vi "1553B-PACKET-1.vi"(8 "数组":u8[](array[numeric])) -> (5 "北向速度":i32, 6 "高度":i32, 7 "纬度":i32, 9 "经度":i32, 10 "系统状态":cluster{"工作状态":string, "工作模式":string}, 11 "真航向":i16, 12 "对准数据来源字":cluster{"位置数据":string, "姿态数据":string}, 13 "横滚角":i16, 14 "组合模式受控状态":cluster{"自动":bool, " 强选":bool}, 15 "俯仰角":i16, 16 "组合数据来源":T7, 17 "地向速度":i32, 18 "组合状态字":T6, 19 "东向速度":i32, 20 "组合导航数据有效字":T1, 21 "GPSBD辅助数据有效字":T5, 22 "系统故障字1":T2, 23 "GLOADSST辅助数据有效字":T4, 24 "北京时间":timestamp, 25 "惯组数据有效字":T3, 26 "单次上电工作时间":i32)   [LabVIEW 2012]
uses:
  index-i32.vi
  index-dbl.vi
  XX-I32.vi
  index-i16.vi
  XX-I16.vi
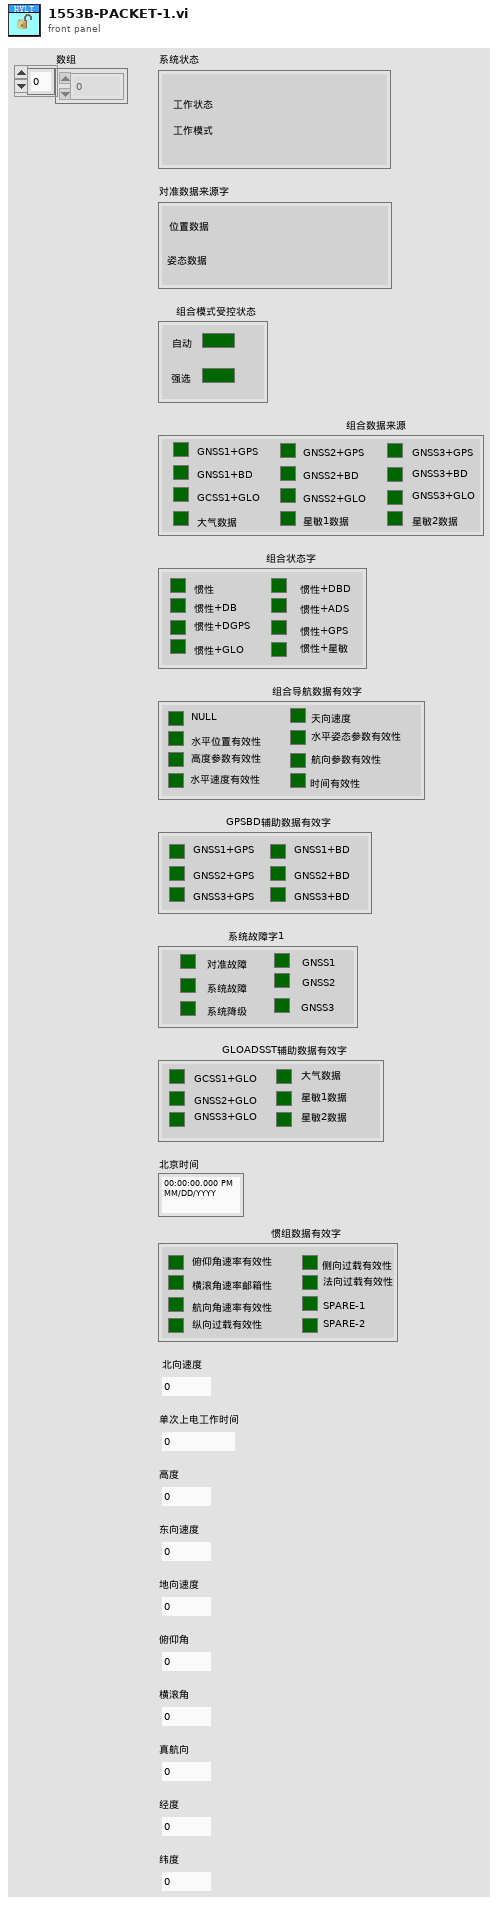
[diagram p1: front panel]
types:
  T1 = cluster{"水平姿态参数有效性":bool, "天向速度":bool, "水平速度有效性":bool, "高度参数有效性":bool, "水平位置有效性":bool, "NULL":bool, " 时间有效性":bool, "航向参数有效性":bool}
  T2 = cluster{"对准故障":bool, "系统故障":bool, "系统降级":bool, "GNSS1":bool, "GNSS2":bool, "GNSS3":bool}
  T3 = cluster{"法向过载有效性":bool, "侧向过载有效性":bool, "纵向过载有效性":bool, "航向角速率有效性":bool, "横滚角速率邮箱性":bool, "俯仰角速率有效性":bool, "SPARE-2":bool, "SPARE-1":bool}
  T4 = cluster{"GCSS1+GLO":bool, "GNSS2+GLO":bool, "GNSS3+GLO":bool, "大气数据":bool, "星敏1数据":bool, "星敏2数据":bool}
  T5 = cluster{"GNSS1+GPS":bool, "GNSS2+GPS":bool, "GNSS2+BD":bool, "GNSS3+BD":bool, "GNSS3+GPS":bool, "GNSS1+BD":bool}
  T6 = cluster{"惯性":bool, "惯性+DGPS":bool, "惯性+DBD":bool, "惯性+GPS":bool, "惯性+DB":bool, "惯性+GLO":bool, "惯性+ADS":bool, "惯性+星敏":bool}
  T7 = cluster{"GNSS1+GPS":bool, "GNSS1+BD":bool, "GCSS1+GLO":bool, "GNSS3+GPS":bool, "GNSS2+GPS":bool, "GNSS2+BD":bool, "GNSS2+GLO":bool, "GNSS3+BD":bool, "GNSS3+GLO":bool, "星敏1数据":bool, "星敏2数据":bool, "大气数据":bool}
  T8 = cluster{"NULL":bool, "水平位置有效性":bool, "高度参数有效性":bool, "水平速度有效性":bool, "天向速度":bool, "水平姿态参数有效性":bool, " 时间有效性":bool, "航向参数有效性":bool}
  T9 = cluster{"俯仰角速率有效性":bool, "横滚角速率邮箱性":bool, "航向角速率有效性":bool, "纵向过载有效性":bool, "侧向过载有效性":bool, "法向过载有效性":bool, "SPARE-2":bool, "SPARE-1":bool}
  T10 = cluster{"GNSS1+GPS":bool, "GNSS1BD":bool, "GNSS3+GPS":bool, "GNSS2+GPS":bool, "GNSS2BD":bool, "GNSS3BD":bool}
  T11 = cluster{"GNSS1+GPS":bool, "GNSS1BD":bool, "GCSS1+GLO":bool, "GNSS3+GPS":bool, "GNSS2+GPS":bool, "GNSS2BD":bool, "GNSS2+GLO":bool, "GNSS3BD":bool, "GNSS3+GLO":bool, "大气数据":bool, "星敏1数据":bool, "星敏2数据":bool}
  T12 = cluster{"组合数据来源[0]":bool, "组合数据来源[1]":bool, "组合数据来源[2]":bool, "组合数据来源[3]":bool, "组合数据来源[4]":bool, "组合数据来源[5]":bool, "组合数据来源[6]":bool, "组合数据来源[7]":bool, "组合数据来源[8]":bool, "组合数据来源[9]":bool, "组合数据来源[10]":bool, "组合数据来源[11]":bool}
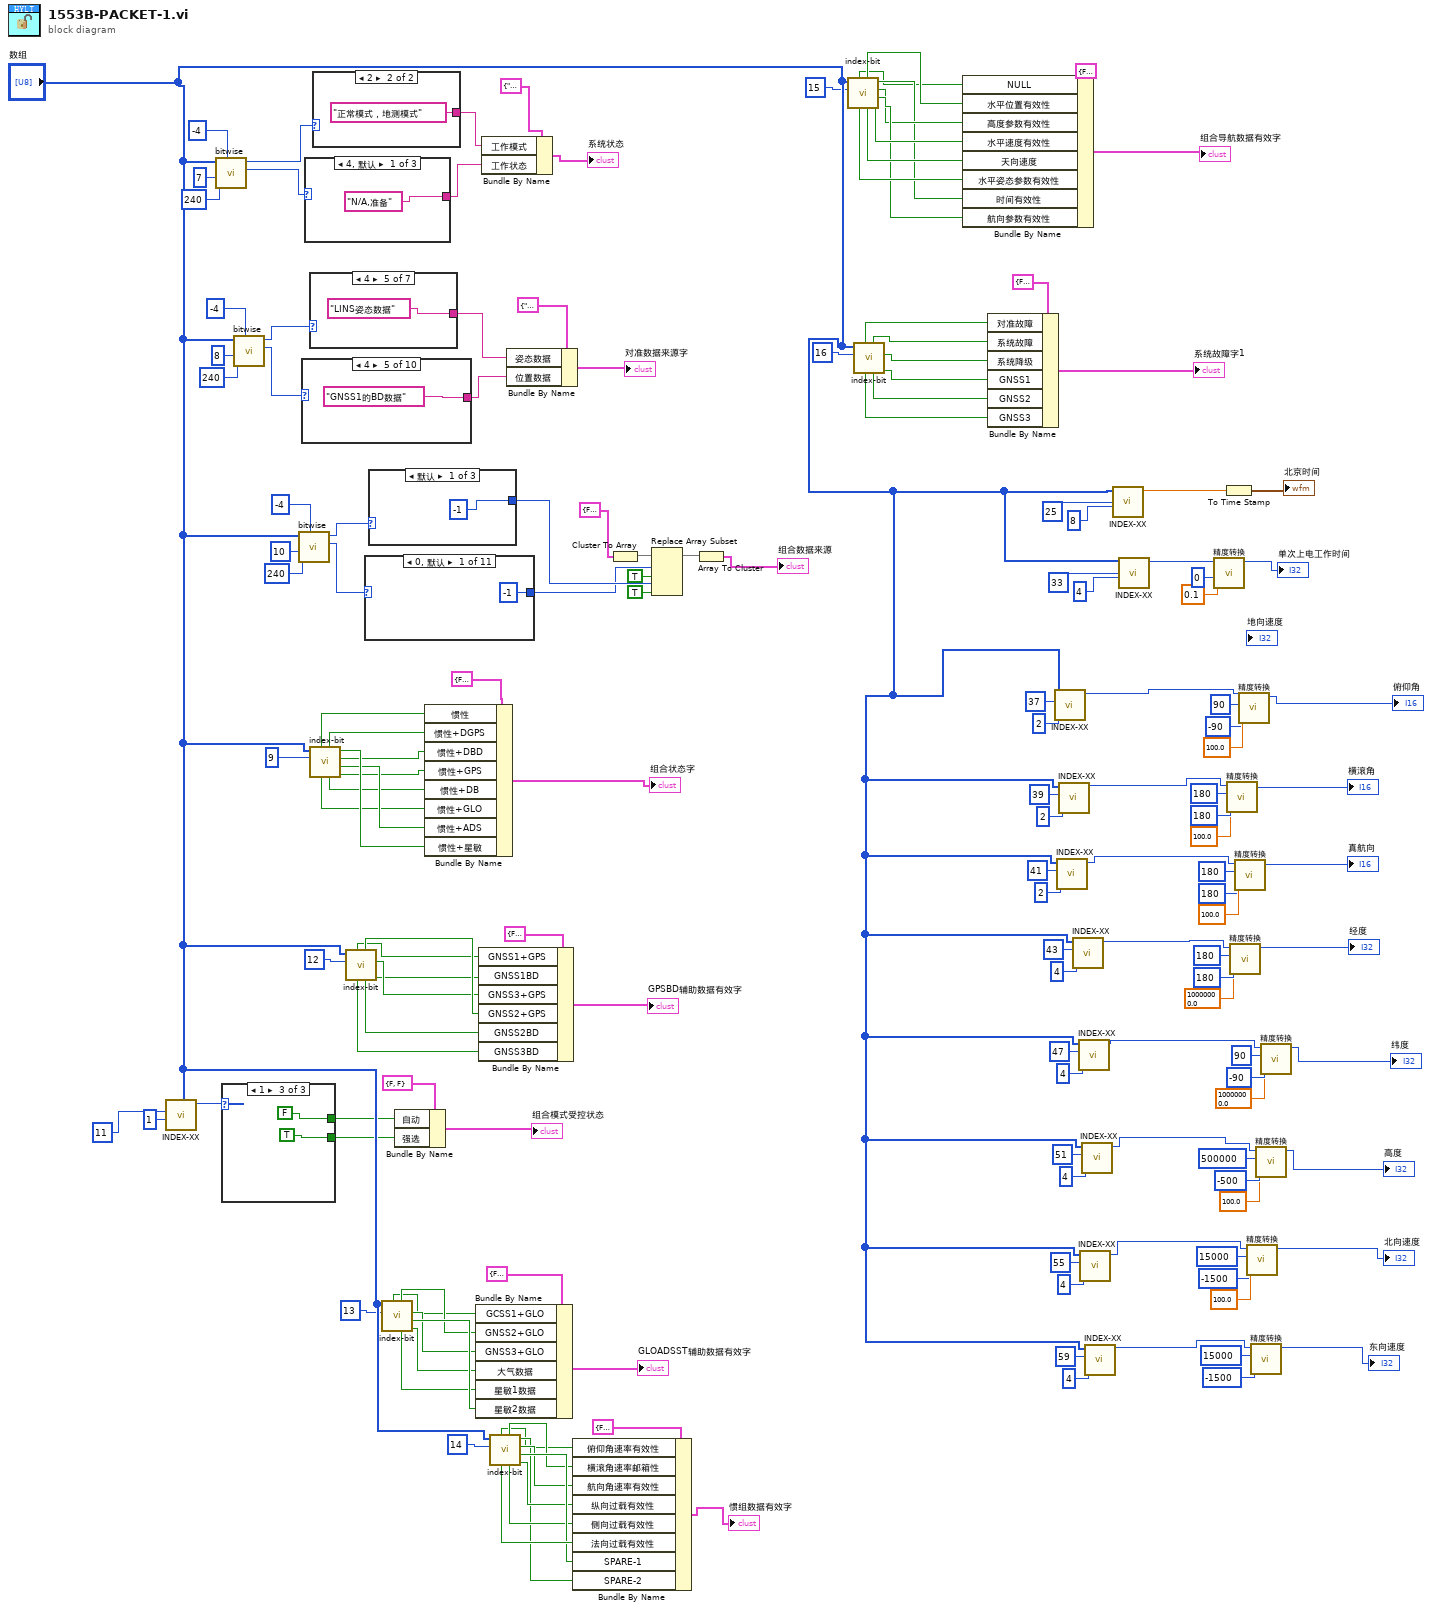
[diagram p0: block diagram]
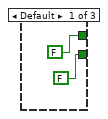
[diagram p2: hidden frame]
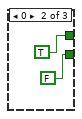
[diagram p3: hidden frame]
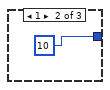
[diagram p4: hidden frame]
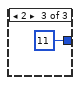
[diagram p5: hidden frame]
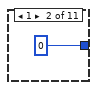
[diagram p6: hidden frame]
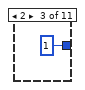
[diagram p7: hidden frame]
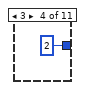
[diagram p8: hidden frame]
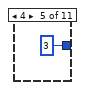
[diagram p9: hidden frame]
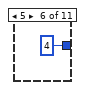
[diagram p10: hidden frame]
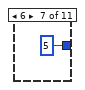
[diagram p11: hidden frame]
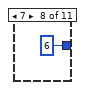
[diagram p12: hidden frame]
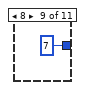
[diagram p13: hidden frame]
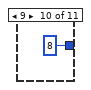
[diagram p14: hidden frame]
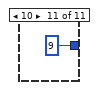
[diagram p15: hidden frame]
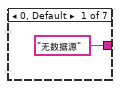
[diagram p16: hidden frame]
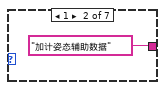
[diagram p17: hidden frame]
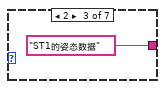
[diagram p18: hidden frame]
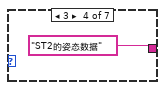
[diagram p19: hidden frame]
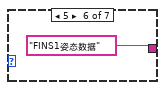
[diagram p20: hidden frame]
diagram:
  n1 = call-poly "INDEX-XX.vi"("长度"=1, "索引"=11, "数组"="数组") -> ("数值输出"=w45:i32)  [unwired: 8 in]
  n2 = call "bitwise.vi"("移位"=i16 -4, "置1"=u8 240, "索引"=7, "数组"="数组") -> ("y2"=w1:u8, "y1"=w2:u8)  [unwired: 6 in]
  n3 = case shown="1" w45 {
    tunnel: [FALSE TRUE FALSE] -> w44
    tunnel: [FALSE FALSE TRUE] -> w43
    frame Default {
    }
    frame 0 {
    }
    frame 1 {
    }
  }
  n4 = call "bitwise.vi"("移位"=i16 -4, "置1"=u8 240, "索引"=8, "数组"="数组") -> ("y2"=w24:u8, "y1"=w23:u8)  [unwired: 6 in]
  n5 = call "bitwise.vi"("移位"=i16 -4, "置1"=u8 240, "索引"=10, "数组"="数组") -> ("y2"=w26:u8, "y1"=w25:u8)  [unwired: 6 in]
  n6 = case shown="4" w24 {
    tunnel: ["无数据源" "GNSS1的GPS数据" "GNSS2的GPS数据" "GNSS3的GPS数据" "GNSS1的BD数据" "GNSS2的BD数据" "GNSS3的BD数据" "GNSS1的GLONASS数据" "GNSS2的GLONASS数据" "GNSS3的GLONASS数据"] -> w6
    frame 0, Default {
    }
    frame 1 {
    }
    frame 2 {
    }
    frame 3 {
    }
    frame 4 {
    }
    frame 5 {
    }
    frame 6 {
    }
    frame 7 {
    }
    frame 8 {
    }
    frame 9 {
    }
  }
  n7 = case shown="4, 默认" w1 {
    tunnel: ["N/A,准备" "罗经对准，在轨对准" "导轨"] -> w3
    frame 4, Default {
    }
    frame 5 {
    }
    frame 6 {
    }
  }
  n8 = case shown="4" w23 {
    tunnel: ["无数据源" "加计姿态辅助数据" "ST1的姿态数据" "ST2的姿态数据" "LINS姿态数据" "FINS1姿态数据" "FINS2姿态数据"] -> w7
    frame 0, Default {
    }
    frame 1 {
    }
    frame 2 {
    }
    frame 3 {
    }
    frame 4 {
    }
    frame 5 {
    }
    frame 6 {
    }
  }
  n9 = call "index-bit.vi"("index"=9 ("索引"), "array"="数组") -> ("bit3"=w34:bool, "bit6"=w37:bool, "bit2"=w33:bool, "bit7"=w38:bool, "bit4"=w35:bool, "bit1"=w32:bool, "bit5"=w36:bool, "bit0"=w31:bool)  [unwired: 2 in]
  n10 = case shown="2" w2 {
    tunnel: ["未知" "正常模式，地测模式"] -> w4
    frame 0, Default {
    }
    frame 2 {
    }
  }
  n11 = call "index-bit.vi"("index"=12 ("索引"), "array"="数组") -> ("bit3"=w52:bool, "bit2"=w53:bool, "bit4"=w55:bool, "bit1"=w54:bool, "bit5"=w56:bool, "bit0"=w51:bool)  [unwired: 2 in, 2 out]
  n12 = case shown="0, 默认" w26 {
    tunnel: [-1 0 1 2 3 4 5 6 7 8 9] -> w10
    frame 0, Default {
    }
    frame 1 {
    }
    frame 2 {
    }
    frame 3 {
    }
    frame 4 {
    }
    frame 5 {
    }
    frame 6 {
    }
    frame 7 {
    }
    frame 8 {
    }
    frame 9 {
    }
    frame 10 {
    }
  }
  n13 = case shown="默认" w25 {
    tunnel: [-1 10 11] -> w13
    frame Default {
    }
    frame 1 {
    }
    frame 2 {
    }
  }
  n14 = call "index-bit.vi"("index"=13 ("索引"), "array"="数组") -> ("bit3"=w64:bool, "bit6"=w66:bool, "bit2"=w63:bool, "bit4"=w65:bool, "bit1"=w62:bool, "bit0"=w61:bool)  [unwired: 2 in, 2 out]
  n15 = Bundle By Name(cluster=cluster{"自动":bool, " 强选":bool} {"自动"=FALSE, " 强选"=FALSE} ("组合模式受控状态"), "自动"=w44, "强选"=w43) -> (→"组合模式受控状态":cluster{"自动":bool, " 强选":bool})
  n16 = Bundle By Name(cluster=T6 {"惯性"=FALSE, "惯性+DGPS"=FALSE, "惯性+DBD"=FALSE, "惯性+GPS"=FALSE, "惯性+DB"=FALSE, "惯性+GLO"=FALSE, "惯性+ADS"=FALSE, "惯性+星敏"=FALSE} ("组合状态"), "惯性"=w31, "惯性+DGPS"=w32, "惯性+DBD"=w33, "惯性+GPS"=w34, "惯性+DB"=w35, "惯性+GLO"=w36, "惯性+ADS"=w37, "惯性+星敏"=w38) -> (→"组合状态字":T6)
  n17 = Bundle By Name(cluster=T4 {"GCSS1+GLO"=FALSE, "GNSS2+GLO"=FALSE, "GNSS3+GLO"=FALSE, "大气数据"=FALSE, "星敏1数据"=FALSE, "星敏2数据"=FALSE} ("GLOADSST辅助数据有效字"), "GCSS1+GLO"=w61, "GNSS2+GLO"=w62, "GNSS3+GLO"=w63, "大气数据"=w64, "星敏1数据"=w65, "星敏2数据"=w66) -> (→"GLOADSST辅助数据有效字":T4)
  n18 = Bundle By Name(cluster=T10 {"GNSS1+GPS"=FALSE, "GNSS1BD"=FALSE, "GNSS3+GPS"=FALSE, "GNSS2+GPS"=FALSE, "GNSS2BD"=FALSE, "GNSS3BD"=FALSE} ("GPSBD辅助数据有效字"), "GNSS1+GPS"=w51, "GNSS1BD"=w52, "GNSS3+GPS"=w53, "GNSS2+GPS"=w54, "GNSS2BD"=w55, "GNSS3BD"=w56) -> (→"GPSBD辅助数据有效字":T10)
  n19 = Bundle By Name(cluster=cluster{"工作状态":string, "工作模式":string} {"工作状态"="", "工作模式"=""} ("系统状态"), "工作模式"=w4, "工作状态"=w3) -> (→"系统状态":cluster{"工作状态":string, "工作模式":string})
  n20 = call "index-bit.vi"("index"=14 ("索引"), "array"="数组") -> ("bit3"=w73:bool, "bit6"=w75:bool, "bit2"=w72:bool, "bit7"=w71:bool, "bit4"=w74:bool, "bit1"=w70:bool, "bit5"=w76:bool, "bit0"=w69:bool)  [unwired: 2 in]
  n21 = Bundle By Name(cluster=cluster{"位置数据":string, "姿态数据":string} {"位置数据"="", "姿态数据"=""} ("数据来源"), "姿态数据"=w7, "位置数据"=w6) -> (→"对准数据来源字":cluster{"位置数据":string, "姿态数据":string})
  n22 = Bundle By Name(cluster=T9 {"俯仰角速率有效性"=FALSE, "横滚角速率邮箱性"=FALSE, "航向角速率有效性"=FALSE, "纵向过载有效性"=FALSE, "侧向过载有效性"=FALSE, "法向过载有效性"=FALSE, "SPARE-2"=FALSE, "SPARE-1"=FALSE} ("惯组数据有效字"), "俯仰角速率有效性"=w69, "横滚角速率邮箱性"=w70, "航向角速率有效性"=w72, "纵向过载有效性"=w73, "侧向过载有效性"=w74, "法向过载有效性"=w76, "SPARE-1"=w75, "SPARE-2"=w71) -> (→"惯组数据有效字":T9)
  n23 = Cluster To Array(cluster=T11 {"GNSS1+GPS"=FALSE, "GNSS1BD"=FALSE, "GCSS1+GLO"=FALSE, "GNSS3+GPS"=FALSE, "GNSS2+GPS"=FALSE, "GNSS2BD"=FALSE, "GNSS2+GLO"=FALSE, "GNSS3BD"=FALSE, "GNSS3+GLO"=FALSE, "大气数据"=FALSE, "星敏1数据"=FALSE, "星敏2数据"=FALSE} ("组合数据来源")) -> (array=w8:bool[])
  n24 = Replace Array Subset(array=w8, new element #1=TRUE ("新元素/子数组"), index #1=w10, new element #2=TRUE ("新元素/子数组"), index #2=w13) -> (w11:bool[])
  n25 = Array To Cluster(array=w11) -> (cluster=→"组合数据来源":T12)
  n26 = call "index-bit.vi"("index"=15 ("索引"), "array"="数组") -> ("bit3"=w86:bool, "bit6"=w85:bool, "bit2"=w84:bool, "bit7"=w83:bool, "bit4"=w87:bool, "bit1"=w82:bool, "bit5"=w88:bool, "bit0"=w81:bool)  [unwired: 2 in]
  n27 = call "index-bit.vi"("index"=16 ("索引"), "array"="数组") -> ("bit3"=w93:bool, "bit2"=w92:bool, "bit4"=w94:bool, "bit1"=w91:bool, "bit5"=w95:bool, "bit0"=w90:bool)  [unwired: 2 in, 2 out]
  n28 = Bundle By Name(cluster=T8 {"NULL"=FALSE, "水平位置有效性"=FALSE, "高度参数有效性"=FALSE, "水平速度有效性"=FALSE, "天向速度"=FALSE, "水平姿态参数有效性"=FALSE, " 时间有效性"=FALSE, "航向参数有效性"=FALSE} ("组合导航数据有效字"), "NULL"=w81, "水平位置有效性"=w82, "高度参数有效性"=w84, "水平速度有效性"=w86, "天向速度"=w87, "水平姿态参数有效性"=w88, "时间有效性"=w83, "航向参数有效性"=w85) -> (→"组合导航数据有效字":T8)
  n29 = Bundle By Name(cluster=T2 {"对准故障"=FALSE, "系统故障"=FALSE, "系统降级"=FALSE, "GNSS1"=FALSE, "GNSS2"=FALSE, "GNSS3"=FALSE} ("系统故障"), "对准故障"=w90, "系统故障"=w91, "系统降级"=w92, "GNSS1"=w93, "GNSS2"=w94, "GNSS3"=w95) -> (→"系统故障字1":T2)
  n30 = call-poly "INDEX-XX.vi"("长度"=2, "索引"=37, "数组"="数组") -> ("数值输出"=w135:i16)  [unwired: 8 in]
  n31 = call-poly "INDEX-XX.vi"("长度"=2, "索引"=41, "数组"="数组") -> ("数值输出"=w127:i16)  [unwired: 8 in]
  n32 = call-poly "INDEX-XX.vi"("长度"=2, "索引"=39, "数组"="数组") -> ("数值输出"=w131:i16)  [unwired: 8 in]
  n33 = call-poly "INDEX-XX.vi"("长度"=4, "索引"=43, "数组"="数组") -> ("数值输出"=w124:i32)  [unwired: 8 in]
  n34 = call-poly "INDEX-XX.vi"("长度"=4, "索引"=47, "数组"="数组") -> ("数值输出"=w116:i32)  [unwired: 8 in]
  n35 = call-poly "INDEX-XX.vi"("长度"=4, "索引"=55, "数组"="数组") -> ("数值输出"=w111:i32)  [unwired: 8 in]
  n36 = call-poly "INDEX-XX.vi"("长度"=4, "索引"=51, "数组"="数组") -> ("数值输出"=w112:i32)  [unwired: 8 in]
  n37 = call-poly "INDEX-XX.vi"("长度"=4, "索引"=59, "数组"="数组") -> ("数值输出"=w108:i32)  [unwired: 8 in]
  n38 = call-poly "INDEX-XX.vi"("长度"=8, "索引"=25, "数组"="数组") -> ("数值输出"=w106:dbl)  [unwired: 8 in]
  n39 = call-poly "INDEX-XX.vi"("长度"=4, "索引"=33, "数组"="数组") -> ("数值输出"=w101:i32)  [unwired: 8 in]
  n40 = call-poly "精度转换.vi"("单位"=0.1, "下限"=0, "数值输入"=w101) -> ("输出"=→"单次上电工作时间":i32)  [unwired: 8 in]
  n41 = To Time Stamp(1:w106) -> (0:→"北京时间":timestamp)
  n42 = call-poly "精度转换.vi"("单位"=100.0, "下限"=i16 180, "上限"=i16 180, "数值输入"=w131) -> ("输出"=→"横滚角":i16)  [unwired: 7 in]
  n43 = call-poly "精度转换.vi"("单位"=10000000.0, "下限"=180, "上限"=180, "数值输入"=w124) -> ("输出"=→"经度":i32)  [unwired: 7 in]
  n44 = call-poly "精度转换.vi"("单位"=100.0, "下限"=i16 180, "上限"=i16 180, "数值输入"=w127) -> ("输出"=→"真航向":i16)  [unwired: 7 in]
  n45 = call-poly "精度转换.vi"("单位"=100.0, "下限"=i16 -90, "上限"=i16 90, "数值输入"=w135) -> ("输出"=→"俯仰角":i16)  [unwired: 7 in]
  n46 = call-poly "精度转换.vi"("单位"=100.0, "下限"=-1500, "上限"=15000, "数值输入"=w111) -> ("输出"=→"北向速度":i32)  [unwired: 7 in]
  n47 = call-poly "精度转换.vi"("下限"=-1500, "上限"=15000, "数值输入"=w108) -> ("输出"=→"东向速度":i32)  [unwired: 8 in]
  n48 = call-poly "精度转换.vi"("单位"=100.0, "下限"=-500, "上限"=500000, "数值输入"=w112) -> ("输出"=→"高度":i32)  [unwired: 7 in]
  n49 = call-poly "精度转换.vi"("单位"=10000000.0, "下限"=-90, "上限"=90, "数值输入"=w116) -> ("输出"=→"纬度":i32)  [unwired: 7 in]
